vi "Launch Nested Models (Mediated).vi"(8 "error in (no error)":errorcluster, 10 "Nested Models":refnum<class "IModel.lvclass">[](array[class]), 11 "IModel in":refnum<class "IModel.lvclass">) -> (0 "error out":errorcluster, 3 "IModel out":refnum<class "IModel.lvclass">)   [LabVIEW 2017, in "IModel.lvlib" / "IModel.lvclass"]
uses:
  IModel.lvclass
  C:/Git/mva-framework/Framework/IObserver/IObserver/IObserver.lvclass
  C:/Program Files (x86)/National Instruments/LabVIEW 2017/vi.lib/ActorFramework/Actor/Actor.lvclass
  IObserver/IObserver/IObserver.lvclass/IObserver.ctl
  IModel.lvclass/IModel.ctl
  <vilib>/ActorFramework/Actor/Actor.lvclass
  IObserver/IObserver/IObserver.lvclass
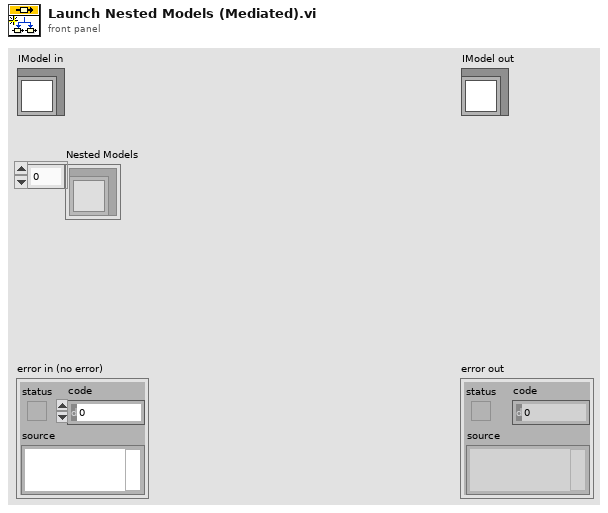
[diagram p1: front panel]
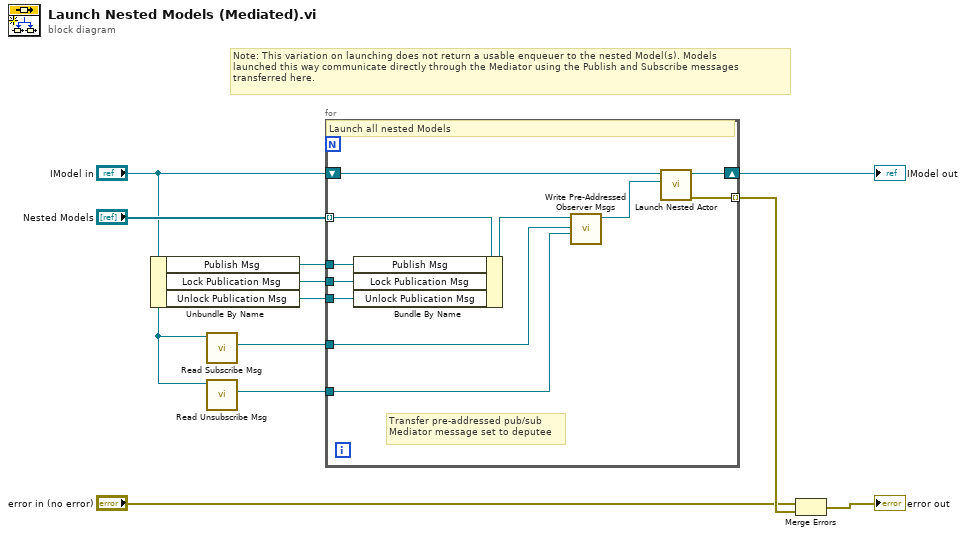
[diagram p0: block diagram]
diagram:
  # "Note: This variation on launching does not return a usable enqueuer to the nested Model(s). Models\nlaunched this way communicate directly through the Mediator using the Publish and Subscribe messages\ntransferred here."
  n1 = Unbundle By Name("IModel in") -> ("Publish Msg"=w6:refnum<class "Publish Msg.lvclass">, "Lock Publication Msg"=w2:refnum<class "Lock Publication Msg.lvclass">, "Unlock Publication Msg"=w1:refnum<class "Unlock Publication Msg.lvclass">)
  n2 = call "Read Subscribe Msg.vi"("IObserver in"="IModel in") -> ("Pre-Addressed Subscribe Msg"=w5:refnum<class "Subscribe Msg.lvclass">)  [unwired: 10 in]
  n3 = call "Read Unsubscribe Msg.vi"("IObserver in"="IModel in") -> ("Pre-Addressed Unsubscribe Msg"=w3:refnum<class "Unsubscribe Msg.lvclass">)  [unwired: 10 in]
  n4 = for {
    shift-right: [w21] -> w11
    shift-left: "IModel in" -> [w22]
    tunnel: "Nested Models" -> [w20] mode=indexing
    tunnel: [w19] -> w9 mode=indexing
    tunnel: w6 -> [w17]
    tunnel: w5 -> [w15]
    tunnel: w3 -> [w14]
    tunnel: w2 -> [w13]
    tunnel: w1 -> [w12]
    # "Transfer pre-addressed pub/sub\nMediator message set to deputee"
    # "Launch all nested Models"
    n5 = Bundle By Name(cluster=w20, "Publish Msg"=w17, "Lock Publication Msg"=w13, "Unlock Publication Msg"=w12) -> (w18:refnum<class "IModel.lvclass">)
    n6 = call "Write Pre-Addressed Observer Msgs.vi"("Pre-Addressed Unsubscribe Msg"=w14, "Pre-Addressed Subscribe Msg"=w15, "IObserver In"=w18) -> ("IObserver Out"=w16:refnum<class "IModel.lvclass">)  [unwired: 8 in]
    n7 = call <vilib>:"Launch Nested Actor.vi"("Nested Actor"=w16, "Caller Actor in"=w22) -> ("error out"=w19:errorcluster, "Caller Actor out"=w21:refnum<class "IModel.lvclass">)  [unwired: 7 in, 1 out]
  }
  "IModel out" <- w11
  n8 = Merge Errors("error in (no error)", w9) -> (→"error out":errorcluster)
